vi "APPLY FIELD.vi"(6 "Numeric in":i32, 7 "Field and Tep  Range":T1={"VISA (Magnet)"="COM4", "Fields(T)"=[], "Temps(K)"=[], "VISA (Temp) "="COM1"}, 8 "error in (no error)":errorcluster, 9 "PSU Status In":T2 {"Trip Current" format="%.3f"; "Trip Field" format="%.4f"; "Voltage" format="%.2f"; "Field Constant" format="%.6f"; "MID Setpoint (T)" format="%.4f"; "MID Setpoint (A)" format="%.3f"; "MAX Setpoint (T)" format="%.4f"; "MAX Setpoint (A)" format="%.3f"; "Heater Voltage" format="%.2f"; "V Limit (V)" format="%.2f"; "Ramp Rate (A/s)" format="%.3f"; "Output (A)" format="%.3f"; "Output (T)" format="%.4f"; "Persistent Current" format="%.3f"; "Persistent Field" format="%.4f"}, 10 "MagQ in":refnum<queue>, 11 "VISA Refnum in":refnum<visa-resource-name>) -> (0 "error out":errorcluster, 1 "PSU Status Out":T2 {"Trip Current" format="%.3f"; "Trip Field" format="%.4f"; "Voltage" format="%.2f"; "Field Constant" format="%.6f"; "MID Setpoint (T)" format="%.4f"; "MID Setpoint (A)" format="%.3f"; "MAX Setpoint (T)" format="%.4f"; "MAX Setpoint (A)" format="%.3f"; "Heater Voltage" format="%.2f"; "V Limit (V)" format="%.2f"; "Ramp Rate (A/s)" format="%.3f"; "Output (A)" format="%.3f"; "Output (T)" format="%.4f"; "Persistent Current" format="%.3f"; "Persistent Field" format="%.4f"}, 2 "MagQ out":refnum<queue>, 3 "VISA Refnum out":refnum<visa-resource-name>, 5 "Numeric out":i32)   [LabVIEW 2025]
uses:
  <instrlib>/SMS LabVIEW Drivers/Source Code/Cryogenic Ltd SMSXXX.lvlib
  <instrlib>/SMS LabVIEW Drivers/Source Code/Public/PSU Status.ctl
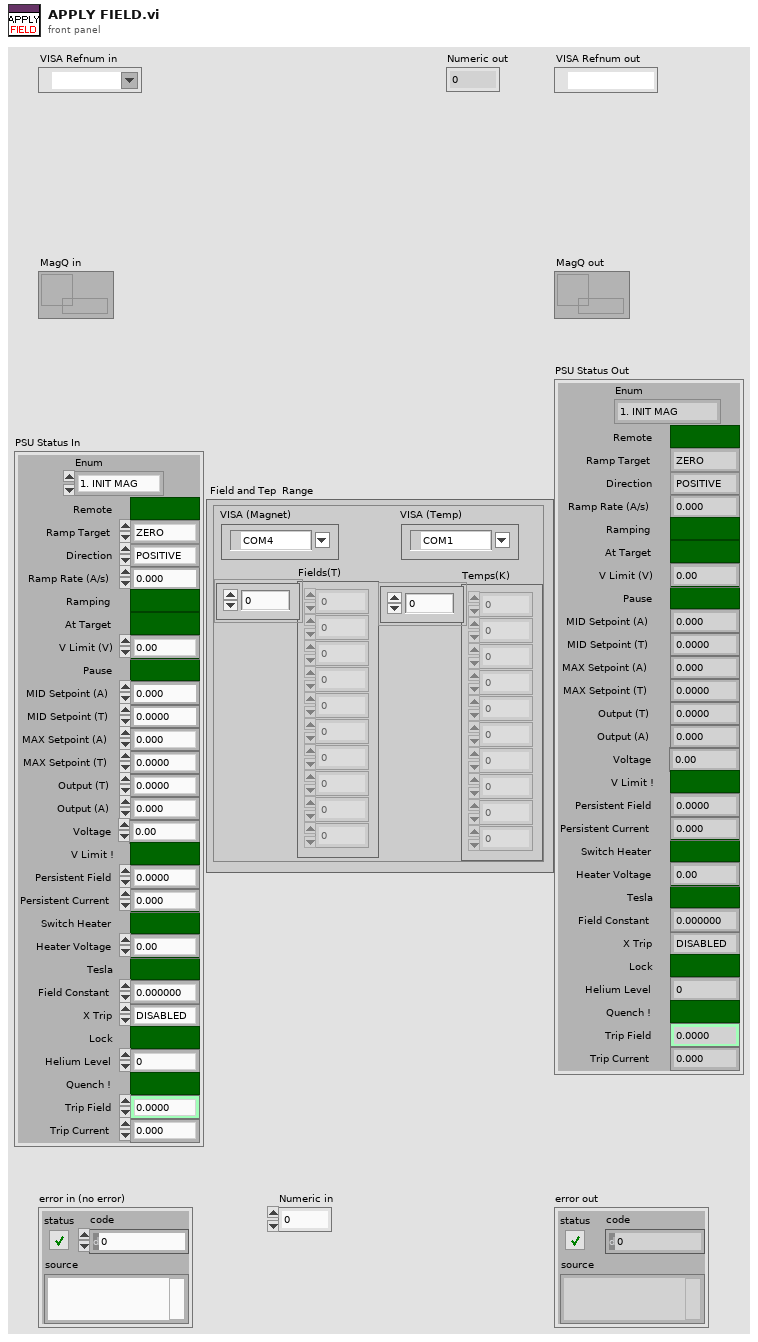
[diagram p1: front panel]
types:
  T1 = cluster{"VISA (Magnet)":refnum<visa-resource-name>, "Fields(T)":dbl[], "Temps(K)":dbl[], "VISA (Temp) ":refnum<visa-resource-name>}
  T2 = typedef "Cryogenic Ltd SMSXXX.lvlib/PSU Status.ctl" = cluster{"Ramp Target":enum16{"ZERO", "MID", "MAX"}, "Pause":bool, "Switch Heater":bool, "Persistent Field":dbl, "Persistent Current":dbl, "Tesla":bool, "Output (T)":dbl, "Output (A)":dbl, "X Trip":enum16{"DISABLED", "ENABLED", "ACTIVE"}, "Ramp Rate (A/s)":dbl, "V Limit (V)":dbl, "Heater Voltage":dbl, "MAX Setpoint (A)":dbl, "MAX Setpoint (T)":dbl, "MID Setpoint (A)":dbl, "MID Setpoint (T)":dbl, "Lock":bool, "Field Constant":dbl, "Remote":bool, "Direction":enum16{"POSITIVE", "NEGATIVE", "OPEN", "UNIPOLAR"}, "Helium Level":u16, "Quench !":bool, "Voltage":dbl, "V Limit !":bool, "Ramping":bool, "At Target":bool, "Trip Field":dbl, "Trip Current":dbl, "Enum":enum16{"1. INIT MAG", "2. MAG ON ", "3. MAG_STAB", "4. MAG IDLE", "5. NEXT FIELD", "6. MAG OFF (Reset)"}}
  T3 = enum16{"1. INIT MAG", "2. MAG ON", "3. MAG_STAB", "4. MAG IDLE", "5. PREP NEXT FIELD", "6. APPLY NEXT FIELD", "7. PREP OFF", "8. MAG OFF (Reset)"}
  T4 = enum16{"RAMP TO ZERO", "RAMP TO MID", "RAMP TO MAX"}
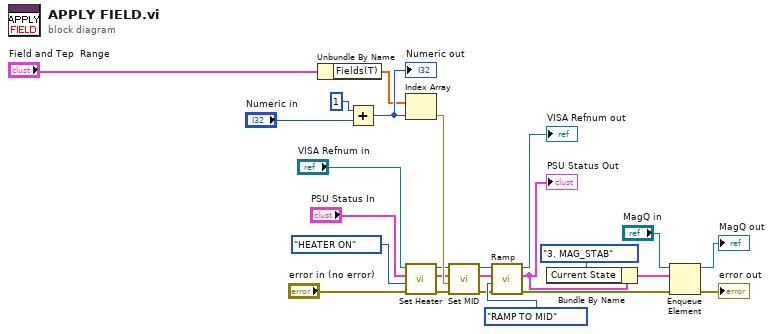
[diagram p0: block diagram]
diagram:
  n1 = Unbundle By Name("Field and Tep  Range") -> ("Fields(T)"=w13:dbl[])
  n2 = Add(x=1, y="Numeric in") -> (x+y=w23:i32)
  "Numeric out" <- w23
  n3 = Index Array(array=w13, index=w23) -> (element=w14:dbl)
  n4 = call <instrlib>:"Set Heater.vi"("Error in (no error)"="error in (no error)", "Heater (On/Off)"=enum16{"HEATER OFF", "HEATER ON"}."HEATER ON", "PSU Status In"="PSU Status In", "VISA Resource Name In"="VISA Refnum in") -> ("Error out"=w6:errorcluster, "PSU Status Out"=w8:T2, "VISA Resource Name Out"=w7:refnum<visa-resource-name>)  [unwired: 4 in, 1 out]
  n5 = call <instrlib>:"Set MID.vi"("Error in (no error)"=w6, "MID (T or A)"=w14, "PSU Status In"=w8, "VISA Resource Name In"=w7) -> ("Error out"=w15:errorcluster, "PSU Status Out"=w16:T2, "VISA Resource Name Out"=w17:refnum<visa-resource-name>)  [unwired: 4 in, 1 out]
  n6 = call <instrlib>:"Ramp.vi"("Error in (no error)"=w15, "Ramp Target"=T4."RAMP TO MID", "PSU Status In"=w16, "VISA Resource Name In"=w17) -> ("Error out"=w24:errorcluster, "PSU Status Out"=w20:T2, "VISA Resource Name Out"=→"VISA Refnum out":refnum<visa-resource-name>)  [unwired: 4 in, 1 out]
  "PSU Status Out" <- w20
  n7 = Bundle By Name(cluster=w20, "Current State"=T3."3. MAG_STAB") -> (w21:T2)
  n8 = Enqueue Element(queue="MagQ in", element=w21, error in (no error)=w24) -> (queue out=→"MagQ out":refnum<queue>, error out=→"error out":errorcluster)  [unwired: 1 in, 1 out]
